vi "Unescape JSON string.vi"(8 "error in (no error)":errorcluster, 11 "Text (with JSON escapes)":string) -> (0 "error out":errorcluster, 3 "Text (unescaped)":string)   [LabVIEW 2024, in "JSONtext.lvlib"]
uses:
  JSONtext.lvlib
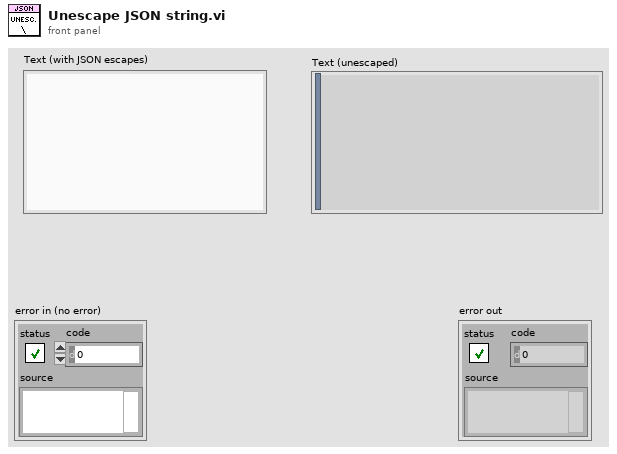
[diagram p1: front panel]
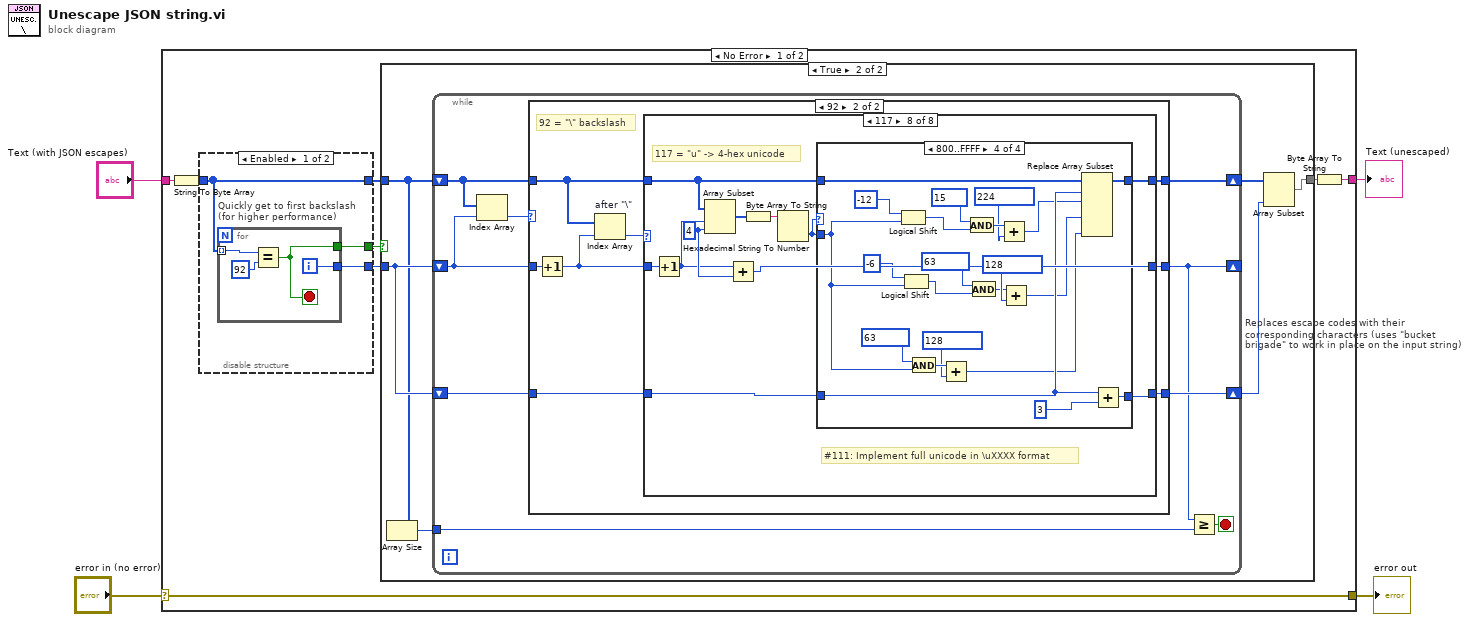
[diagram p0: block diagram]
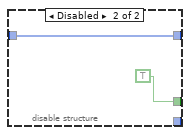
[diagram p2: hidden frame]
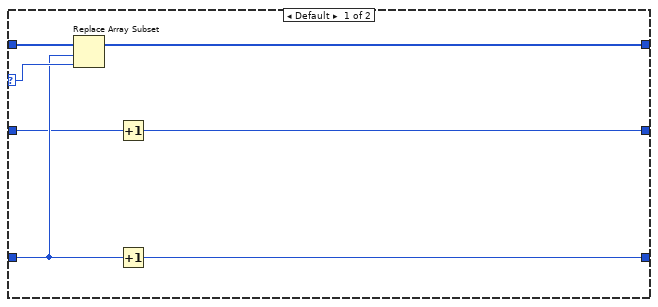
[diagram p4: hidden frame]
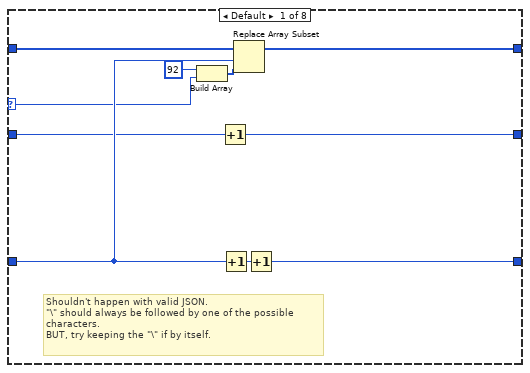
[diagram p5: hidden frame]
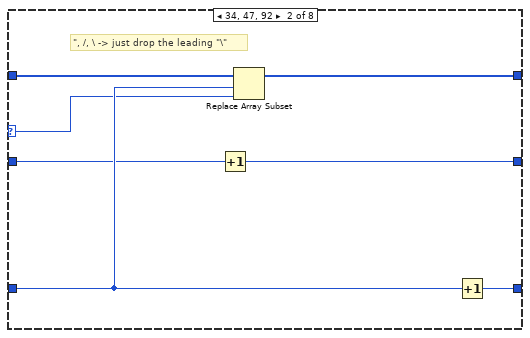
[diagram p6: hidden frame]
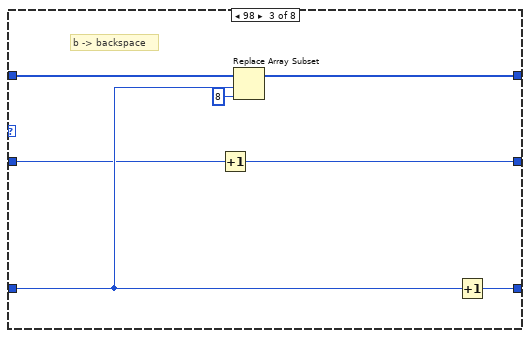
[diagram p7: hidden frame]
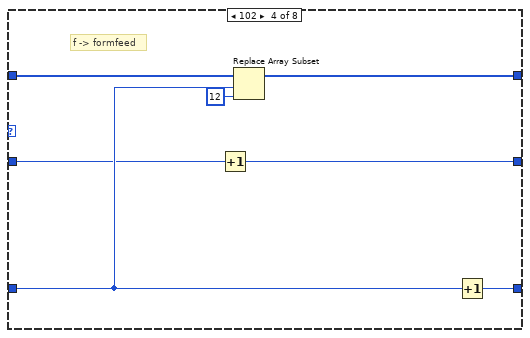
[diagram p8: hidden frame]
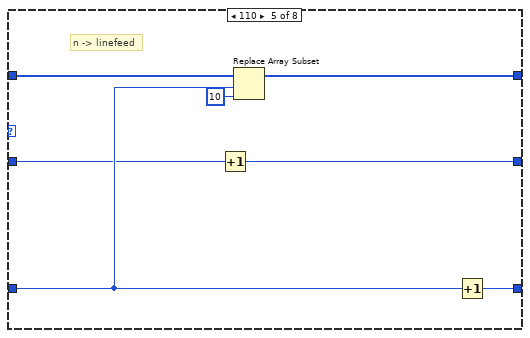
[diagram p9: hidden frame]
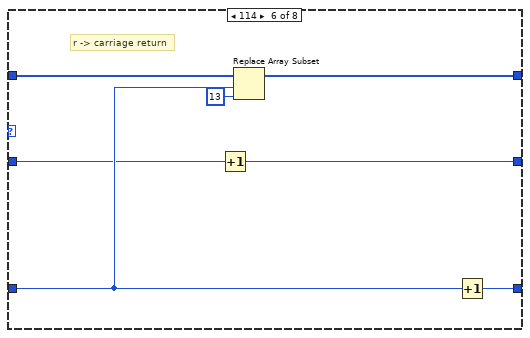
[diagram p10: hidden frame]
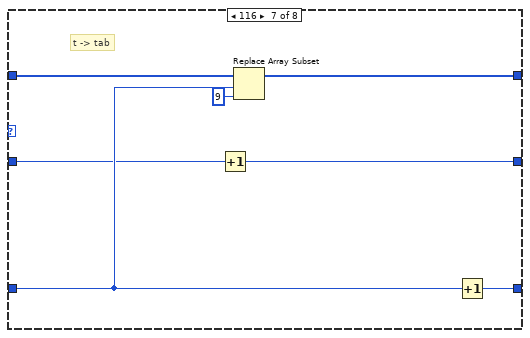
[diagram p11: hidden frame]
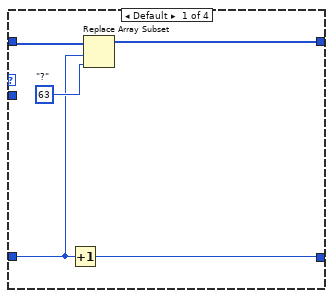
[diagram p12: hidden frame]
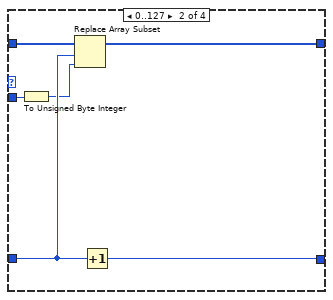
[diagram p13: hidden frame]
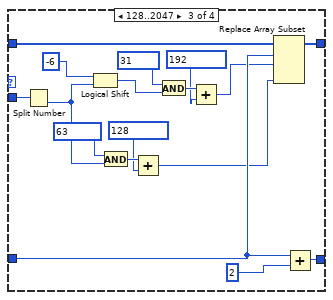
[diagram p14: hidden frame]
diagram:
  n1 = case shown="No Error" "error in (no error)" {
    selector: "error in (no error)" -> [w12 w167]
    tunnel: [w12 w167] -> w3
    tunnel: "Text (with JSON escapes)" -> [w11 w166]
    tunnel: [w9 w166] -> w1
    frame No Error {
      n2 = String To Byte Array(string=w11) -> (unsigned byte array=w8:u8[])
      n3 = disable-structure shown="Enabled" {
        disable-tunnel: w8 -> [w13 w21]
        disable-tunnel: [w15 _] -> w7
        disable-tunnel: [w13 w21] -> w6
        disable-tunnel: [w14 TRUE] -> w5
        frame Enabled {
          n4 = for "Quickly get to first backslash\n(for higher performance)" {
            tunnel: w13 -> [w18] mode=indexing
            tunnel: [w17] -> w15
            tunnel: [w16] -> w14
            i -> [w17]
            stop <- w16 stop-if-true
            n5 = Equal?(x=w18, y=u8 92 ("new element/subarray")) -> (x = y?=w16:bool)
          }
        }
        frame Disabled {
        }
      }
      n6 = case shown="True" w5 {
        tunnel: [w22 w26] -> w10
        tunnel: w7 -> [_ w24]
        tunnel: w6 -> [w22 w23]
        frame False {
          # "No escapes in string"
        }
        frame True {
          n7 = Array Size(array=w23) -> (size(s)=w25:i32)
          n8 = while "Replaces escape codes with their corresponding characters (uses \"bucket brigade\" to work in place on the input string)" {
            shift-right: [w33] -> w28
            shift-left: w23 -> [w36]
            shift-right: [w30] -> _
            shift-left: w24 -> [w35]
            shift-right: [w32] -> w27
            shift-left: w24 -> [w34]
            tunnel: w25 -> [w29]
            stop <- w31 stop-if-true
            n9 = Index Array(array=w36, index=w35) -> (element=w37:u8)
            n10 = case shown="92" w37 {
              selector: w37 -> [w43 _]
              tunnel: w36 -> [w44 w50]
              tunnel: w35 -> [w40 w51]
              tunnel: w34 -> [w41 w47]
              tunnel: [w42 w48] -> w33
              tunnel: [w39 w45] -> w32
              tunnel: [w38 w46] -> w30
              frame Default {
                n11 = Replace Array Subset(array=w44, new element=w43, index=w41) -> (w42:u8[])
                n12 = Increment(x=w40) -> (x+1=w38:i32)
                n13 = Increment(x=w41) -> (x+1=w39:i32)
              }
              frame 92 {
                # "92 = \"\\\" backslash"
                n14 = Increment(x=w51) -> (x+1=w49:i32)
                n15 = Index Array "after \"\\\""(array=w50, index=w49) -> (element=w52:u8)
                n16 = case shown="117" w52 {
                  selector: w52 -> [w54 w63 _ _ _ _ _ _]
                  tunnel: w50 -> [w62 w69 w76 w83 w90 w97 w104 w106]
                  tunnel: w49 -> [w57 w65 w72 w79 w86 w93 w100 w113]
                  tunnel: [w61 w68 w75 w82 w89 w96 w103 w105] -> w48
                  tunnel: w47 -> [w58 w66 w73 w80 w87 w94 w101 w108]
                  tunnel: [w56 w64 w71 w78 w85 w92 w99 w111] -> w46
                  tunnel: [w53 w67 w74 w81 w88 w95 w102 w107] -> w45
                  frame Default {
                    # "Shouldn't happen with valid JSON.  \n\"\\\" should always be followed by one of the possible\ncharacters.\nBUT, try keeping the \"\\\" if by itself."
                    n17 = Build Array(u8 92 ("new element/subarray"), w54) -> (w55:u8[])
                    n18 = Increment(x=w57) -> (x+1=w56:i32)
                    n19 = Increment(x=w58) -> (x+1=w59:i32)
                    n20 = Replace Array Subset(array=w62, new element=w55, index=w58) -> (w61:u8[])
                    n21 = Increment(x=w59) -> (x+1=w53:i32)
                  }
                  frame 34, 47, 92 {
                    # "\", /, \\ -> just drop the leading \"\\\""
                    n22 = Increment(x=w65) -> (x+1=w64:i32)
                    n23 = Replace Array Subset(array=w69, new element=w63, index=w66) -> (w68:u8[])
                    n24 = Increment(x=w66) -> (x+1=w67:i32)
                  }
                  frame 98 {
                    # "b -> backspace"
                    n25 = Increment(x=w72) -> (x+1=w71:i32)
                    n26 = Replace Array Subset(array=w76, new element=u8 8 ("new element/subarray"), index=w73) -> (w75:u8[])
                    n27 = Increment(x=w73) -> (x+1=w74:i32)
                  }
                  frame 102 {
                    # "f -> formfeed"
                    n28 = Increment(x=w79) -> (x+1=w78:i32)
                    n29 = Replace Array Subset(array=w83, new element=u8 12 ("new element/subarray"), index=w80) -> (w82:u8[])
                    n30 = Increment(x=w80) -> (x+1=w81:i32)
                  }
                  frame 110 {
                    # "n -> linefeed"
                    n31 = Increment(x=w86) -> (x+1=w85:i32)
                    n32 = Replace Array Subset(array=w90, new element=u8 10 ("new element/subarray"), index=w87) -> (w89:u8[])
                    n33 = Increment(x=w87) -> (x+1=w88:i32)
                  }
                  frame 114 {
                    # "r -> carriage return"
                    n34 = Increment(x=w93) -> (x+1=w92:i32)
                    n35 = Replace Array Subset(array=w97, new element=u8 13 ("new element/subarray"), index=w94) -> (w96:u8[])
                    n36 = Increment(x=w94) -> (x+1=w95:i32)
                  }
                  frame 116 {
                    # "t -> tab"
                    n37 = Increment(x=w100) -> (x+1=w99:i32)
                    n38 = Replace Array Subset(array=w104, new element=u8 9 ("new element/subarray"), index=w101) -> (w103:u8[])
                    n39 = Increment(x=w101) -> (x+1=w102:i32)
                  }
                  frame 117 {
                    w112 = 4 ("length")
                    # "#111: Implement full unicode in \\uXXXX format"
                    # "117 = \"u\" -> 4-hex unicode"
                    n40 = Increment(x=w113) -> (x+1=w110:i32)
                    n41 = Array Subset(array=w106, index=w110, length=w112) -> (w115:u8[])
                    n42 = Add(x=w110, y=w112) -> (x+y=w111:i32)
                    n43 = Byte Array To String(unsigned byte array=w115) -> (string=w114:string)
                    n44 = Hexadecimal String To Number(string=w114) -> (number=w109:u32)  [unwired: 2 in, 1 out]
                    n45 = case shown="800..FFFF" w109 {
                      tunnel: w109 -> [_ w126 w138 w150]
                      tunnel: w108 -> [w117 w123 w139 w161]
                      tunnel: [w116 w125 w143 w165] -> w107
                      tunnel: w106 -> [w119 w124 w141 w163]
                      tunnel: [w120 w121 w142 w164] -> w105
                      frame Default {
                        w118 = u8 63  # "?"
                        n46 = Increment(x=w117) -> (x+1=w116:i32)
                        n47 = Replace Array Subset(array=w119, new element=w118, index=w117) -> (w120:u8[])
                      }
                      frame 0..127 {
                        n48 = To Unsigned Byte Integer(number=w126) -> (unsigned 8bit integer=w122:u8)
                        n49 = Replace Array Subset(array=w124, new element=w122, index=w123) -> (w121:u8[])
                        n50 = Increment(x=w123) -> (x+1=w125:i32)
                      }
                      frame 128..2047 {
                        n51 = Split Number(x=w138) -> (lo(x)=w127:u16)  [unwired: 1 out]
                        n52 = Logical Shift(y=i16 -6, x=w127) -> (x << y=w131:u16)
                        n53 = And(x=u16 63, y=w127) -> (x .and. y?=w136:u16)
                        n54 = Add(x=w136, y=u16 128 ("x")) -> (x+y=w128:u16)
                        n55 = And(x=u16 31, y=w131) -> (x .and. y?=w133:u16)
                        n56 = Add(x=w133, y=u16 192 ("x")) -> (x+y=w129:u16)
                        n57 = Replace Array Subset(array=w141, new element #1=w129, index #1=w139, new element #2=w128) -> (w142:u8[])  [unwired: 1 in]
                        n58 = Add(x=w139, y=2) -> (x+y=w143:i32)
                      }
                      frame 2048..65535 {
                        n59 = Logical Shift(y=i16 -12, x=w150) -> (x << y=w154:u32)
                        n60 = Logical Shift(y=i16 -6, x=w150) -> (x << y=w146:u32)
                        n61 = And(x=u32 63, y=w150) -> (x .and. y?=w159:u32)
                        n62 = Add(x=w159, y=u32 128 ("x")) -> (x+y=w145:u32)
                        n63 = And(x=u32 15, y=w154) -> (x .and. y?=w156:u32)
                        n64 = And(x=u32 63, y=w146) -> (x .and. y?=w148:u32)
                        n65 = Add(x=w156, y=u32 224 ("x")) -> (x+y=w152:u32)
                        n66 = Add(x=w148, y=u32 128 ("x")) -> (x+y=w144:u32)
                        n67 = Replace Array Subset(array=w163, new element #1=w152, index #1=w161, new element #2=w144, new element #3=w145) -> (w164:u8[])  [unwired: 2 in]
                        n68 = Add(x=w161, y=3) -> (x+y=w165:i32)
                      }
                    }
                  }
                }
              }
            }
            n69 = Greater Or Equal?(x=w30, y=w29) -> (x >= y?=w31:bool)
          }
          n70 = Array Subset(array=w28, length=w27) -> (w26:u8[])  [unwired: 1 in]
        }
      }
      n71 = Byte Array To String(unsigned byte array=w10) -> (string=w9:string)
    }
    frame Error {
    }
  }
  "error out" <- w3
  "Text (unescaped)" <- w1
